vi "Sensor_data_to_value.vi"(10 "Sensor data":u16, 11 "Sensor type":u8 format="%x") -> (2 "Signal legend":string, 3 "Value ouptut":dbl)   [LabVIEW 2013]
doc: "Converts sensor type data to human readable value format\nADC to mV\nLight sensor to Lux\nTemperature to [10*degC]\nRelative humidity to [10*%RH]"
panel:
  # "Converts sensor type data to human readable value format\nADC to mV\nLight sensor to Lux\nTemperature to [10*degC]\nRelative humidity to [10*%RH]"
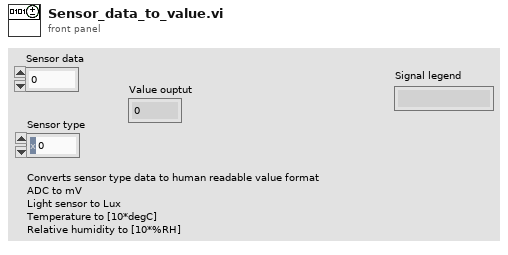
[diagram p1: front panel]
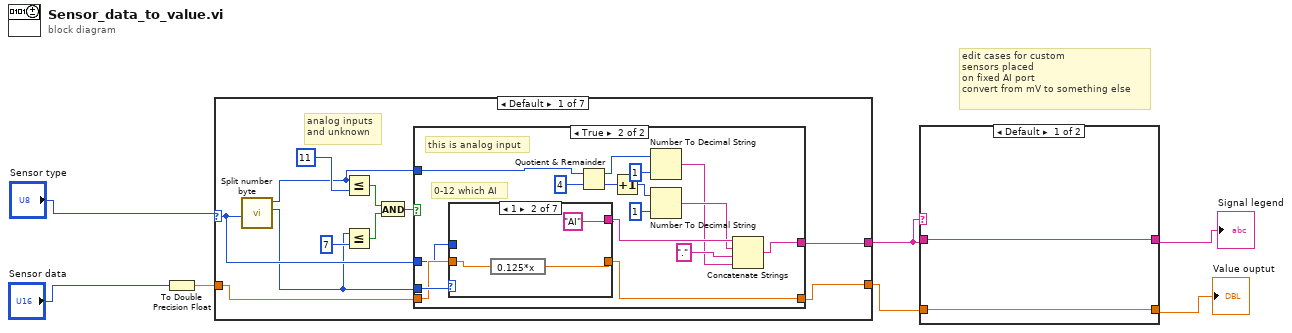
[diagram p0: block diagram]
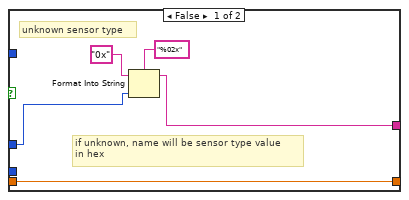
[diagram p3: hidden frame]
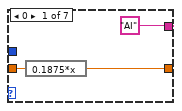
[diagram p4: hidden frame]
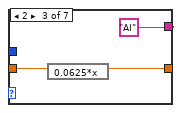
[diagram p5: hidden frame]
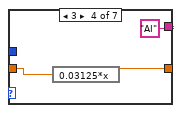
[diagram p6: hidden frame]
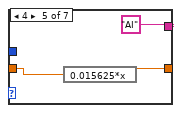
[diagram p7: hidden frame]
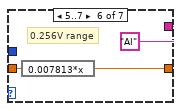
[diagram p8: hidden frame]
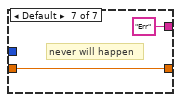
[diagram p9: hidden frame]
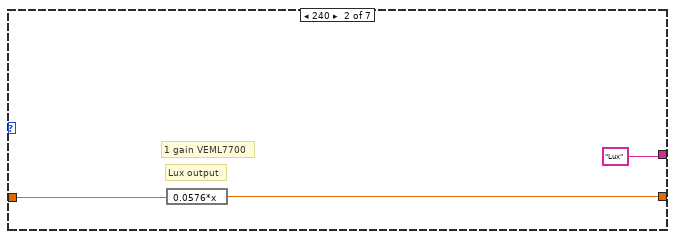
[diagram p10: hidden frame]
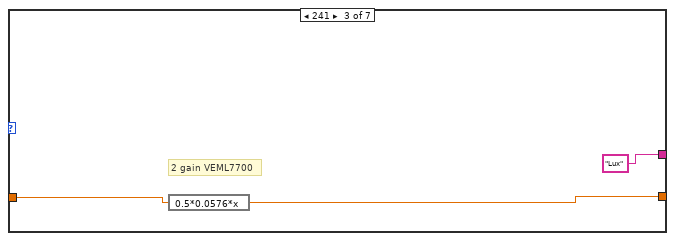
[diagram p11: hidden frame]
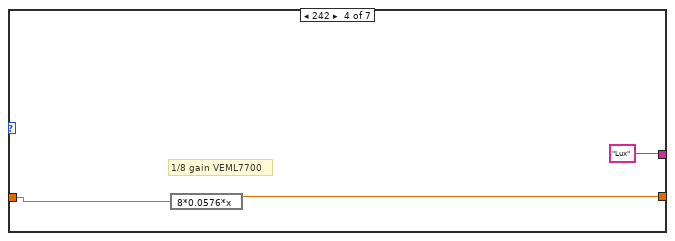
[diagram p12: hidden frame]
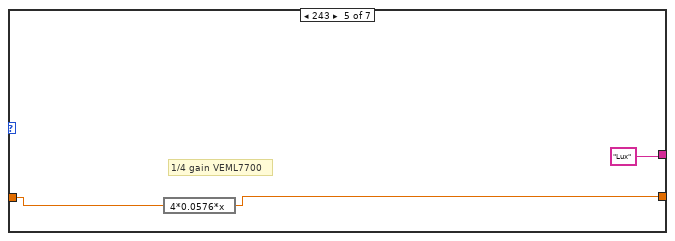
[diagram p13: hidden frame]
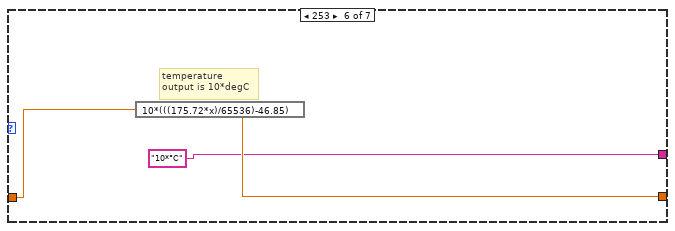
[diagram p14: hidden frame]
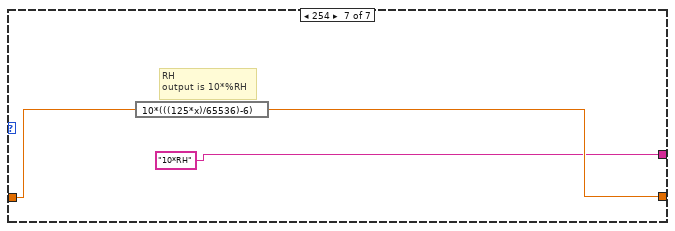
[diagram p15: hidden frame]
diagram:
  # "edit cases for custom \nsensors placed\non fixed AI port\nconvert from mV to something else"
  n1 = To Double Precision Float(number="Sensor data") -> (double precision float=w6:dbl)
  n2 = case shown="Default" "Sensor type" {
    selector: "Sensor type" -> [w10 _ _ _ _ _ _]
    tunnel: w6 -> [w12 w62 w65 w68 w71 w74 w77]
    tunnel: [w11 w61 w64 w67 w70 w73 w76] -> w5
    tunnel: [w13 "Lux" ("initial string") "Lux" ("initial string") "Lux" ("initial string") "Lux" ("initial string") "10*°C" ("initial string") "10*RH" ("initial string")] -> w1
    frame Default {
      # "analog inputs\nand unknown"
      n3 = call "Split number byte.vi"("x"=w10) -> ("lo(x)"=w9:u8, "hi(x)"=w8:u8)  [unwired: 9 in]
      n4 = Less Or Equal?(x=w8, y=u8 11) -> (x <= y?=w16:bool)
      n5 = Less Or Equal?(x=w9, y=u8 7) -> (x <= y?=w15:bool)
      n6 = And(x=w16, y=w15) -> (x .and. y?=w14:bool)
      n7 = case shown="True" w14 {
        tunnel: w9 -> [_ w39]
        tunnel: w10 -> [w21 w37]
        tunnel: [w20 w30] -> w13
        tunnel: w12 -> [w19 w38]
        tunnel: [w19 w29] -> w11
        tunnel: w8 -> [_ w25]
        frame False {
          # "if unknown, name will be sensor type value\nin hex"
          # "unknown sensor type"
          n8 = Format Into String(format string="%02x", initial string="0x", w21) -> (resulting string=w20:string)  [unwired: 1 in, 1 out]
        }
        frame True {
          # "0-12 which AI"
          # "this is analog input"
          n9 = case shown="1" w39 {
            tunnel: [w42 w45 w48 w51 w54 w57 w59] -> w29
            tunnel: ["AI" ("initial string") "AI" ("initial string") "AI" ("initial string") "AI" ("initial string") "AI" ("initial string") "AI" ("initial string") "Err" ("initial string")] -> w32
            tunnel: w38 -> [w40 w43 w46 w49 w52 w55 w59]
            tunnel: w37 -> [_ _ _ _ _ _ _]
            frame 0 {
              n10 = expression code="0.1875*x"(w40) -> (w42:dbl)
            }
            frame 1 {
              n11 = expression code="0.125*x"(w43) -> (w45:dbl)
            }
            frame 2 {
              n12 = expression code="0.0625*x"(w46) -> (w48:dbl)
            }
            frame 3 {
              n13 = expression code="0.03125*x"(w49) -> (w51:dbl)
            }
            frame 4 {
              n14 = expression code="0.015625*x"(w52) -> (w54:dbl)
            }
            frame 5..7 {
              # "0.256V range"
              n15 = expression code="0.007813*x"(w55) -> (w57:dbl)
            }
            frame Default {
              # "never will happen"
            }
          }
          n16 = Quotient & Remainder(x=w25, y=u8 4) -> (x-y*floor(x/y)=w26:u8, floor(x/y)=w35:u8)
          n17 = Increment(x=w35) -> (x+1=w24:u8)
          n18 = Number To Decimal String(number=w26, width (-)=i16 1) -> (decimal integer string=w27:string)
          n19 = Number To Decimal String(number=w24, width (-)=i16 1) -> (decimal integer string=w28:string)
          n20 = Concatenate Strings(w32, w28, "." ("string"), w27) -> (w30:string)
        }
      }
    }
    frame 240 {
      # "Lux output"
      # "1 gain VEML7700"
      n21 = expression code="0.0576*x"(w62) -> (w61:dbl)
    }
    frame 241 {
      # "2 gain VEML7700"
      n22 = expression code="0.5*0.0576*x"(w65) -> (w64:dbl)
    }
    frame 242 {
      # "1/8 gain VEML7700"
      n23 = expression code="8*0.0576*x"(w68) -> (w67:dbl)
    }
    frame 243 {
      # "1/4 gain VEML7700"
      n24 = expression code="4*0.0576*x"(w71) -> (w70:dbl)
    }
    frame 253 {
      # "temperature\noutput is 10*degC"
      n25 = expression code="10*(((175.72*x)/65536)-46.85)"(w74) -> (w73:dbl)
    }
    frame 254 {
      # "RH\noutput is 10*%RH"
      n26 = expression code="10*(((125*x)/65536)-6)"(w77) -> (w76:dbl)
    }
  }
  n27 = case shown="Default" w1 {
    tunnel: w5 -> [w79 w81]
    tunnel: [w79 w81] -> w4
    tunnel: [w78 w80] -> w3
    tunnel: w1 -> [w78 w80]
    frame Default {
    }
    frame "A1.0" {
    }
  }
  "Value ouptut" <- w4
  "Signal legend" <- w3
